vi "CMI.vi"() -> ()   [LabVIEW 2013]
panel:
  out "AMI码波形图":i8[](graph)
  in  "停止":bool
  in  "计数":u8
  out "变换后的AM码":i8[](array[numeric])
  in  "原消息代码":u32[](array[numeric])
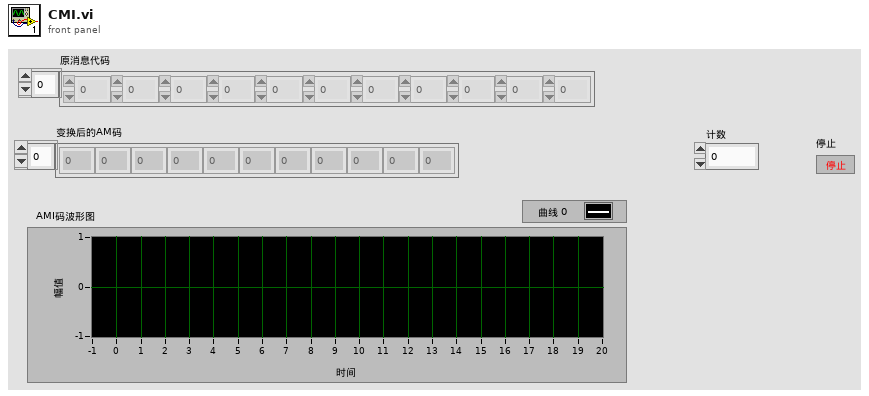
[diagram p1: front panel]
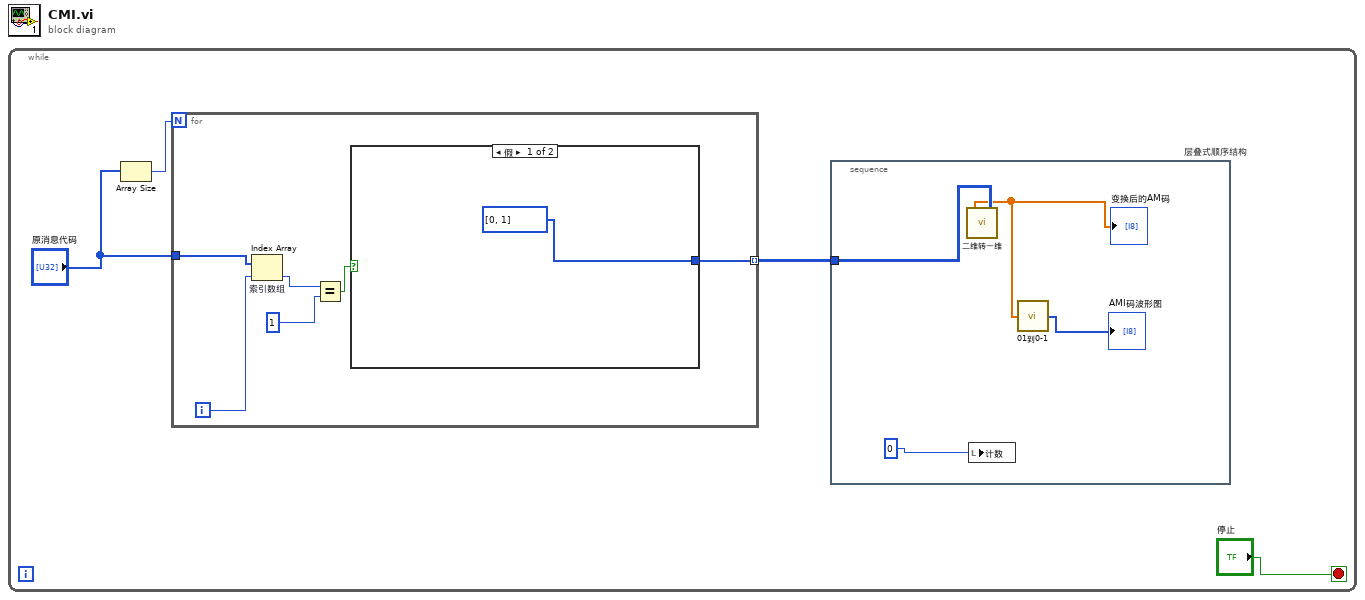
[diagram p0: block diagram]
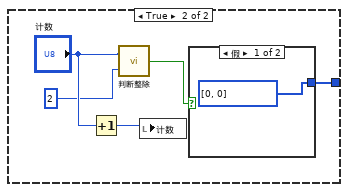
[diagram p2: hidden frame]
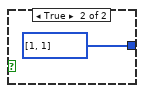
[diagram p3: hidden frame]
diagram:
  n1 = while {
    stop <- "停止" stop-if-true
    n2 = Array Size(array="原消息代码") -> (size(s)=w2:i32)
    n3 = for {
      N: w2 -> [_]
      tunnel: [w14] -> w3 mode=indexing
      tunnel: "原消息代码" -> [w12]
      i -> [w11]
      n4 = Index Array "索引数组"(array=w12, index=w11) -> (element=w10:u32)
      n5 = Equal?(x=w10, y=1) -> (x = y?=w13:bool)
      n6 = case shown="假" w13 {
        tunnel: [i32[] [0, 1] w16] -> w14
        frame False {
        }
        frame True {
          n7 = Increment(x="计数") -> (x+1=w17:u8)
          n8 = call "判断整除.vi"("被除数"=2, "除数"="计数") -> ("布尔"=w18:bool)
          n9 = local write "计数"(w17) -> ()
          n10 = case shown="假" w18 {
            tunnel: [i32[] [0, 0] i32[] [1, 1]] -> w16
            frame False {
            }
            frame True {
            }
          }
        }
      }
    }
    n11 = stacked-sequence "层叠式顺序结构" {
      tunnel: w3 -> [w7]
      frame #0 {
        n12 = call "二维转一维.vi"("输入2维"=w7) -> ("输出一维"=w6:dbl[])
        "变换后的AM码" <- w6
        n13 = local write "计数"(0) -> ()
        n14 = call "01到0-1.vi"("1,0码元"=w6) -> ("1，-1码元"=→"AMI码波形图":i8[])
      }
    }
  }
